vi "Read Execution time.vi"(11 "Test Suite Result In":T1) -> (1 "Execution time string":string, 2 "Execution time":dbl, 3 "Test Suite Result Out":T1)   [LabVIEW 2020, in "Test Suite Result.lvlib"]
uses:
  Test Suite Result.lvlib
  Test Suite Result.ctl
  Core/Result/Status.ctl
  Case Result/Test Case Result.ctl
  Method Result/Method Result.ctl
  Assertion Result/Assertion Result.ctl
  Assertion Result/Public/TypeDefs/Assertion Type.ctl
  Assertion Result/Assertion Result.lvlib
  Method Result/Method Result.lvlib
  Case Result/Test Case Result.lvlib
  Core/Result/Result.lvlib
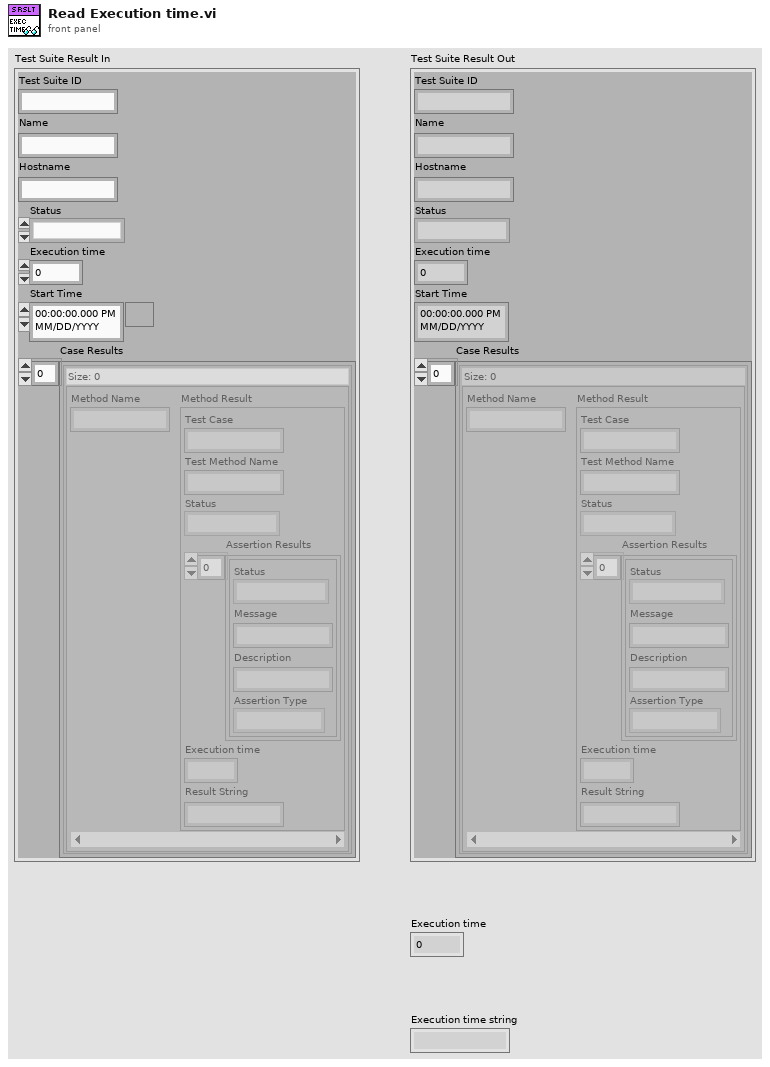
[diagram p1: front panel]
types:
  T1 = typedef "Test Suite Result.lvlib/Test Suite Result.ctl" = cluster{"Test Suite ID":string, "Name":string, "Hostname":string, "Status":T2, "Execution time":dbl, "Start Time":timestamp, "Case Results":T3[]}
  T2 = typedef "Result.lvlib/Status.ctl" = enum16{"", "Passed", "Failed", "Error", "Skipped", "Setup Error", "Broken", "Teardown Error"}
  T3 = typedef "Test Case Result.lvlib/Test Case Result.ctl" = map{string, T4}
  T4 = typedef "Method Result.lvlib/Method Result.ctl" = cluster{"Test Case":string, "Test Method Name":string, "Status":T2, "Assertion Results":T5[], "Execution time":dbl, "Result String":string}
  T5 = typedef "Assertion Result.lvlib/Assertion Result.ctl" = cluster{"Status":T2, "Message":string, "Description":string, "Assertion Type":T6}
  T6 = typedef "Result.lvlib/Assertion Type.ctl" = enum16{"None", "Pass", "Fail", "Skip", "Pass if Equal", "Fail if Equal", "Pass if Error", "Fail if Error", "Pass if", "Fail if"}
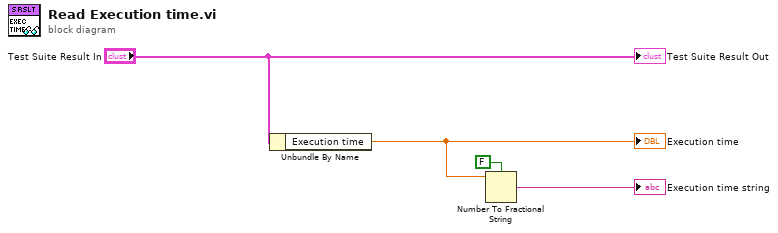
[diagram p0: block diagram]
diagram:
  n1 = Unbundle By Name("Test Suite Result In") -> ("Execution time"=w1:dbl)
  "Execution time" <- w1
  n2 = Number To Fractional String(use system decimal point (T)=FALSE, number=w1) -> (F-format string=→"Execution time string":string)  [unwired: 2 in]
  "Test Suite Result Out" <- "Test Suite Result In"
